vi "Actor Core.vi"(8 "error in":errorcluster, 11 "File Reader in":refnum<class "File Reader.lvclass">) -> (0 "error out":errorcluster, 3 "Actor out":refnum<class "Actor.lvclass">)   [LabVIEW 2020, in "File Reader.lvlib" / "File Reader.lvclass"]
doc: "(<B>Filename</B>: Actor Framework.lvlib:Actor.lvclass:Actor Core.vi)\n\nReceives messages to the actor, reacts to them, and initiates any error handling that may shut the actor down.\n\nDescendant classes may override this VI to append parallel tasks for the actor to complete while it handles messages. Overrides use the Call Parent Method node."
uses:
  File Reader.lvclass
  C:/Users/AlexK/work/LabVIEW Programme/HIJ_Vision_Project/Submodules/HIJ Vision/Camera Actors/Camera Actor/Camera Actor/Camera Actor.lvclass
  C:/Program Files (x86)/National Instruments/LabVIEW 2020/vi.lib/ActorFramework/Actor/Actor.lvclass
  <vilib>/ActorFramework/Actor/Actor.lvclass
  Camera Actor/Camera Actor/Camera Actor.lvclass/Camera Actor.ctl
  <vilib>/ActorFramework/Actor/Actor.lvclass/Actor.ctl
  <vilib>/ActorFramework/Message Enqueuer/Message Enqueuer.lvclass/Message Enqueuer.ctl
  Camera Actor/Camera Actor Messages/Publish Image Msg/Publish Image Msg.lvclass/Publish Image Msg.ctl
  <vilib>/numeric/Random Number (Range) U64.vi
  Camera Actor/Camera Actor/Write Camera Name.vi
  <vilib>/numeric/sub_Random U32.vi
  <vilib>/ActorFramework/Message Enqueuer/Init from Existing Queue.vi
  <vilib>/ActorFramework/Message Enqueuer/Enqueue.vi
  Camera Actor/Camera Actor Messages/Publish Image Msg/Publish Image Msg.lvclass
  C:/Program Files (x86)/National Instruments/LabVIEW 2020/vi.lib/ActorFramework/Message/Message.lvclass
  <vilib>/ActorFramework/Message Priority Queue/Priority Enqueue.vi
  Camera Actor/Camera Actor/Camera Actor.lvclass
  <vilib>/ActorFramework/Message Enqueuer/Message Enqueuer.lvclass
panel:
  in  "Stop Button":bool
  in  "Image File":path=path "C:/Users/AlexK/work/LabVIEW Programme/Test/for yasmina/9,9qm q=0,43_A2 q=0,43  A=9,9 µm2 _cam6 201602-10 14.05.55.png"
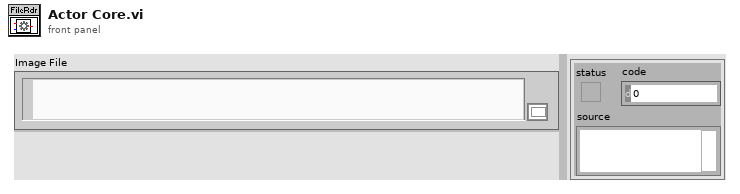
[diagram p1: front panel]
types:
  T1 = typedef "Image Type" = u32
  T2 = enum32{"Invalid", "Standard", "Closed", "Hidden", "Minimized", "Maximized"}
  T3 = typedef "IMAQ Image.ctl" = refnum<image>
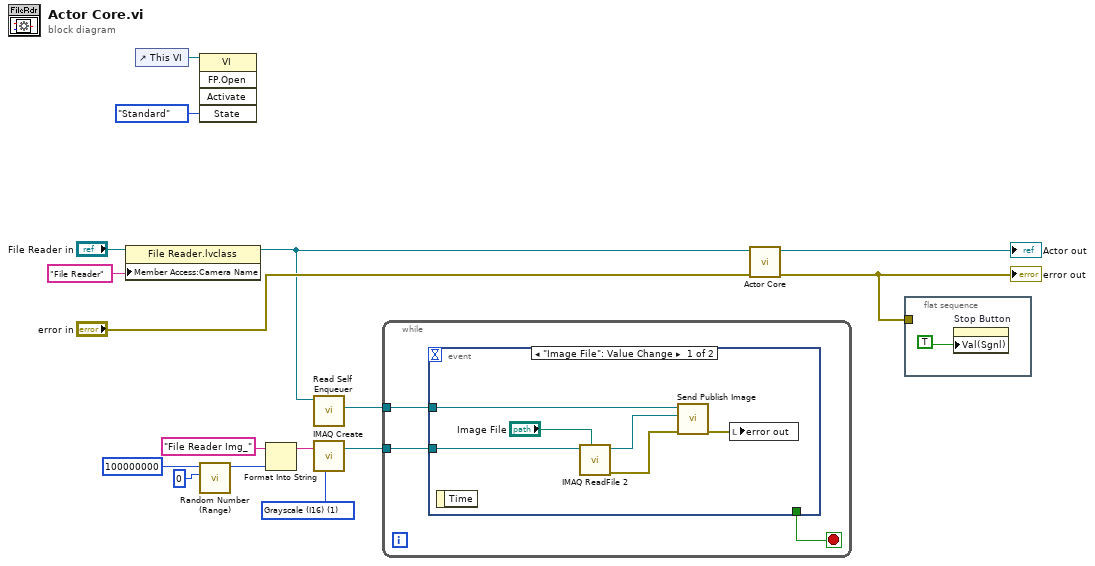
[diagram p0: block diagram]
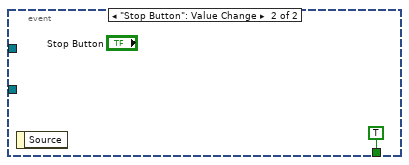
[diagram p2: hidden frame]
diagram:
  w9 = T1 1 items=["Grayscale (U8)", "Grayscale (I16)", "Grayscale (SGL)", "Complex (CSG)", "RGB (U32)", "HSL (U32)", "RGB (U64)", "Grayscale (U16)"] ("Image Type")
  n1 = property class="File Reader.lvclass"(reference="File Reader in", "Member Access:Camera Name"="File Reader" ("Camera Name")) -> (reference out=w2:refnum<class "File Reader.lvclass">)  [unwired: 1 in, 1 out]
  n2 = control-ref of="This VI"() -> (w13:refnum<vi>)
  n3 = invoke class="VI" method="FP.Open"(reference=w13, "State"=T2."Standard" ("Front Panel Window:State")) -> ()  [unwired: 3 in, 5 out]
  n4 = call-poly <vilib>:"Random Number (Range).vi"("lower bound (0)"=u64 0, "upper bound (100)"=u64 100000000) -> ("number"=w6:u64)  [unwired: 9 in]
  n5 = Format Into String(initial string="File Reader Img_" ("Image Name"), w6) -> (resulting string=w7:string)  [unwired: 2 in, 1 out]
  n6 = call <vilib>:"Read Self Enqueuer.vi"("Actor"=w2) -> ("Self Enqueuer"=w10:refnum<class "Message Enqueuer.lvclass">)  [unwired: 10 in]
  n7 = call "IMAQ Create"("Image Name"=w7, "Image Type"=w9) -> ("New Image"=w3:T3)  [unwired: 3 in, 1 out]
  n8 = while {
    tunnel: w10 -> [w19]
    tunnel: w3 -> [w18]
    stop <- w17 stop-if-true
    n9 = event shown="[0] \"Image File\": Value Change" {
      selector: _ -> [_ _]
      dyn-events: _ -> [_ _]
      timeout: _ -> [_ _]
      tunnel: w19 -> [w25 _]
      tunnel: w18 -> [w24 _]
      tunnel: [_ TRUE ("Stop Button")] -> w17
      event "Image File": Value Change {
        n10 = event-data() -> ()  [unwired: 1 in, 1 out]
        n11 = call "IMAQ ReadFile 2"("File Path"="Image File", "Image"=w24) -> ("error out"=w21:errorcluster, "Image Out"=w22:T3)  [unwired: 5 in, 3 out]
        n12 = call "Send Publish Image.vi"("error in (no error)"=w21, "Image"=w22, "Message Enqueuer"=w25) -> ("error out"=w20:errorcluster)  [unwired: 7 in, 1 out]
        n13 = local write "error out"(w20) -> ()
      }
      event "Stop Button": Value Change {
        n14 = event-data() -> ()  [unwired: 1 in, 1 out]
      }
    }
  }
  n15 = call-parent "Actor Core.vi"("error in"="error in", "Camera Actor in"=w2) -> ("error out"=w11:errorcluster, "Actor out"=→"Actor out":refnum<class "Actor.lvclass">)  [unwired: 8 in]
  "error out" <- w11
  n16 = flat-sequence {
    tunnel: w11 -> [_]
    frame #0 {
      n17 = property on="Stop Button" class="Bool (strict)"("Val(Sgnl)"=TRUE) -> ()  [unwired: 2 in, 2 out]
    }
  }
